vi "4 probe data-osc-time v1.5.vi"() -> ()   [LabVIEW 2014]
uses:
  <vilib>/Analysis/baseanly.llb/Mean (DBL).vi
  <instrlib>/Tektronix TDS 200 1000 2000 Series/Tektronix TDS 200 1000 2000 Series.lvlib
  <vilib>/Analysis/NI_AALBase.lvlib
panel:
  out "Seconds":sgl
  in  "stop button":bool
  in  "loop num":dbl=10000000000.0
  out "Data IV Keithley":string
  in  "Data IV Keithley 2":path=path "c:/myfile.txt"
  out "IV Curve":cluster{dbl[], i32[]}(graph)
  in  "Stop Button":bool
  out "Ch1":dbl
  out "Ch2":dbl
  out "Ch3":dbl
  out "Ch4":dbl
  in  "Channel 4 (3: Channel 4)":u16(ring)=3 items=["Channel 1", "Channel 2", "Channel 3", "Channel 4", "Math", "Reference A", "Reference B", "Reference C", "Reference D"]
  in  "Probe Attenuation 4 (0.1)":dbl=0.1
  in  "Vertical Coupling 4 (1: DC)":u16(ring)=1 items=["AC", "DC", "Ground"]
  in  "Channel 3 (2: Channel 3)":u16(ring)=2 items=["Channel 1", "Channel 2", "Channel 3", "Channel 4", "Math", "Reference A", "Reference B", "Reference C", "Reference D"]
  in  "Probe Attenuation 3 (0.1)":dbl=0.1
  in  "Vertical Coupling 3 (1: DC)":u16(ring)=1 items=["AC", "DC", "Ground"]
  in  "Channel 2 (1: Channel 2)":u16(ring)=1 items=["Channel 1", "Channel 2", "Channel 3", "Channel 4", "Math", "Reference A", "Reference B", "Reference C", "Reference D"]
  in  "Channel 1 (0: Channel 1)":u16(ring) items=["Channel 1", "Channel 2", "Channel 3", "Channel 4", "Math", "Reference A", "Reference B", "Reference C", "Reference D"]
  in  "Serial Configuration":T1={"Baud Rate"=9600, "Parity"=0, "Stop Bits"=10, "Flow Control"=2} {"Flow Control" items=["None", "XON/XOFF", "RTS/CTS", "XON/XOFF & RTS/CTS", "DTR/DSR", "XON/XOFF & DTR/DSR"]; "Stop Bits" items=["1.0"=10, "1.5"=15, "2.0"=20]; "Parity" items=["None", "Odd", "Even", "Mark", "Space"]; "Baud Rate" items=["300"=300, "600"=600, "1200"=1200, "2400"=2400, "4800"=4800, "9600"=9600, "19200"=19200]}
  in  "Probe Attenuation 2 (0.1)":dbl=0.1
  in  "Vertical Coupling 2 (1: DC)":u16(ring)=1 items=["AC", "DC", "Ground"]
  in  "Probe Attenuation 1 (0.1)":dbl=0.1
  in  "Vertical Coupling 1 (1: DC)":u16(ring)=1 items=["AC", "DC", "Ground"]
  in  "Timeout (10000 ms)":u32=500
  in  "VISA resource name":refnum<visa-resource-name>="USB0::0x0699::0x03A6::C044157::INSTR"
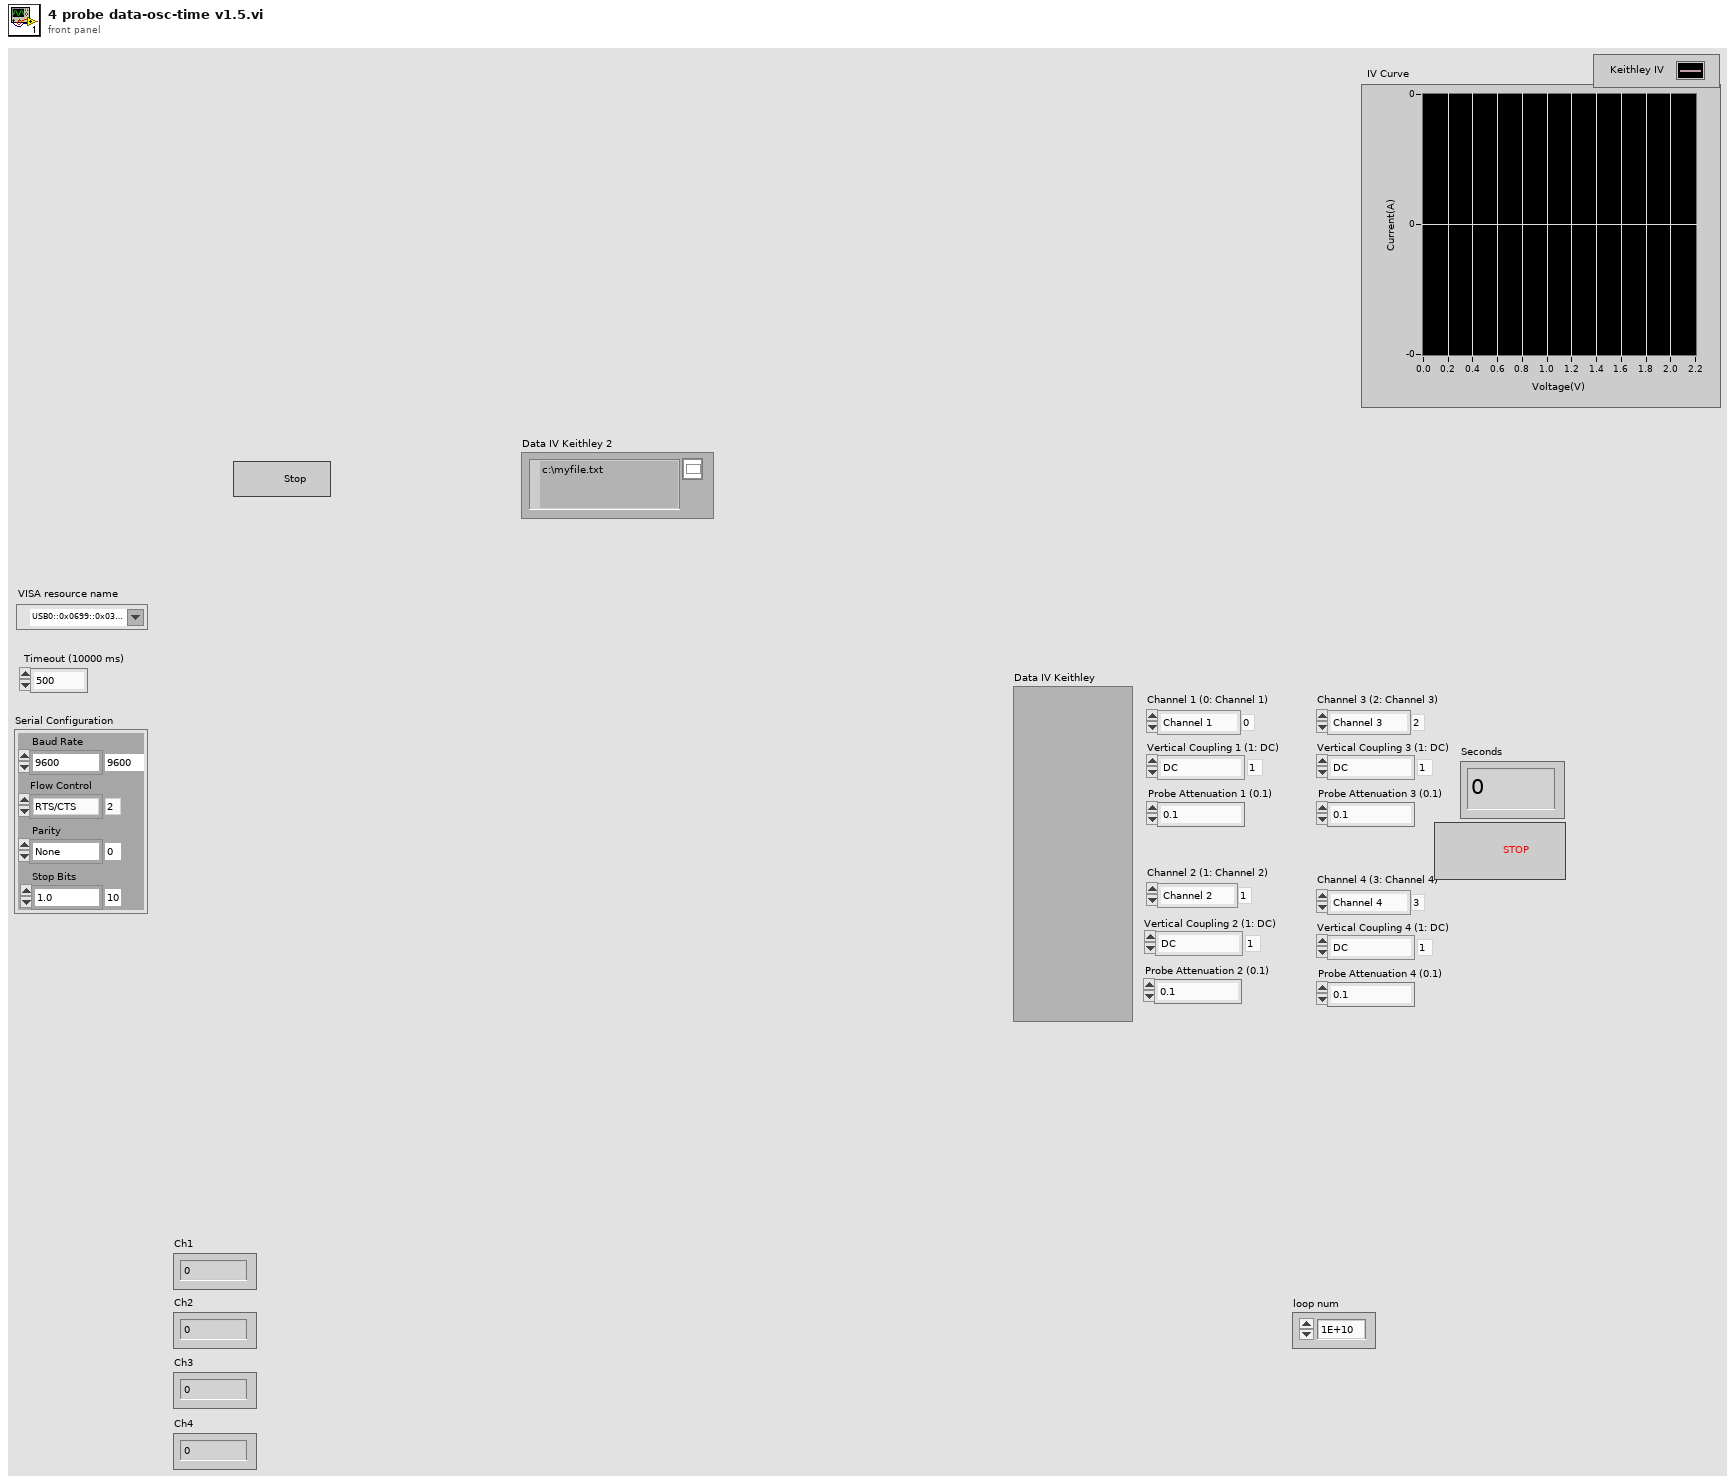
[diagram p1: front panel]
types:
  T1 = cluster{"Baud Rate":u32, "Parity":u16, "Stop Bits":u16, "Flow Control":u16}
  T2 = enum16{"open", "replace", "create", "open or create", "replace or create", "replace or create with confirmation"}
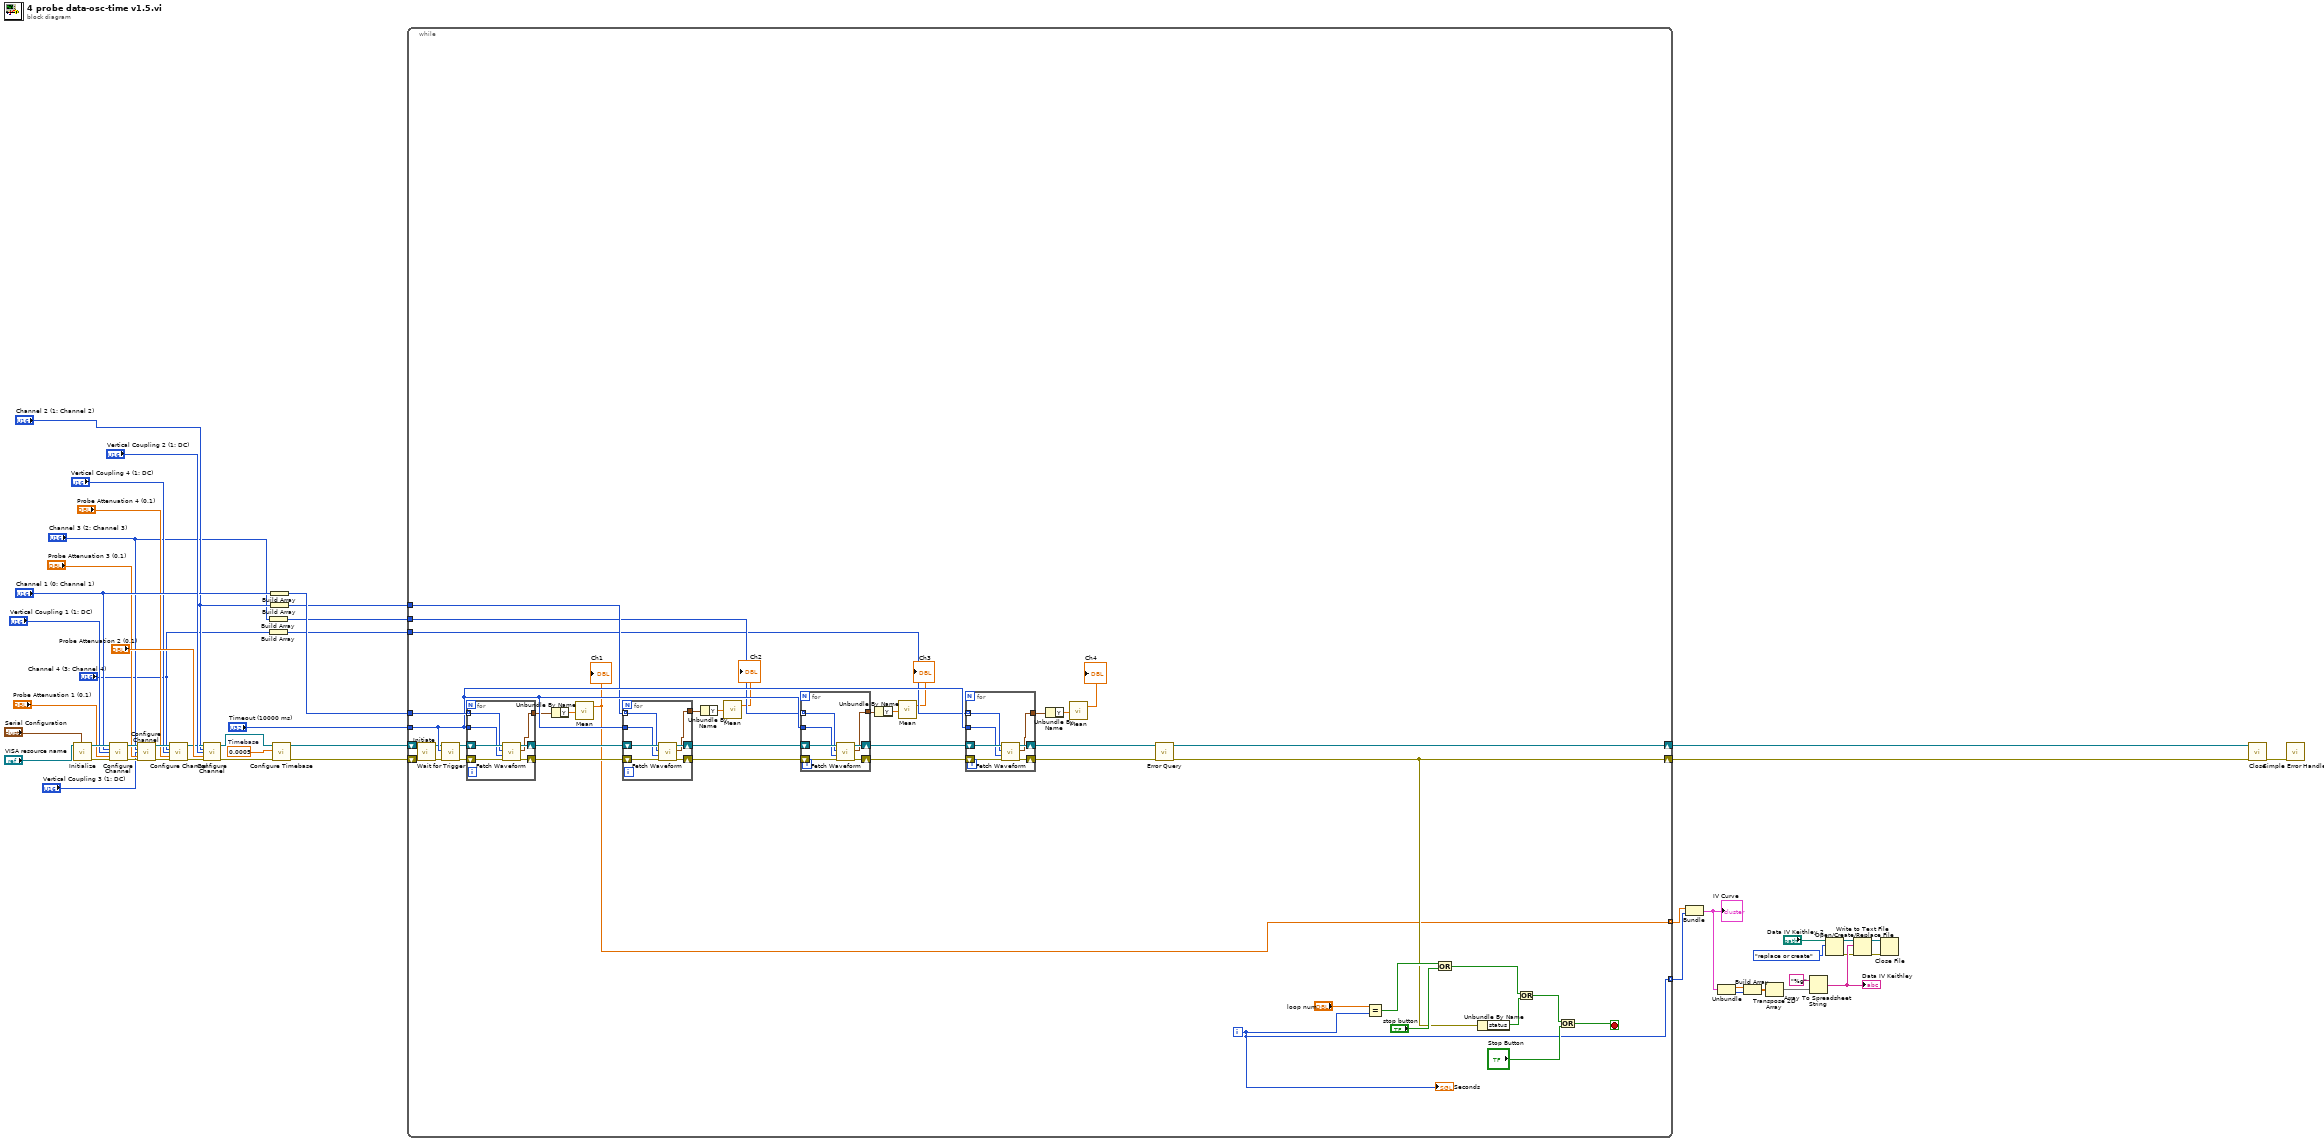
[diagram p0: block diagram]
diagram:
  w36 = 0.0005  # Timebase
  n1 = call <instrlib>:"Initialize.vi"("Serial Configuration"="Serial Configuration", "VISA resource name"="VISA resource name") -> ("error out"=w45:errorcluster, "VISA resource name out"=w46:refnum<visa-resource-name>)  [unwired: 3 in, 5 out]
  n2 = call <instrlib>:"Configure Channel.vi"("VISA resource name"=w46, "Channel (0: Channel 1)"="Channel 1 (0: Channel 1)", "Vertical Coupling (1: DC)"="Vertical Coupling 1 (1: DC)", "Probe Attenuation (10: 10X)"="Probe Attenuation 1 (0.1)", "error in (no error)"=w45) -> ("VISA resource name out"=w31:refnum<visa-resource-name>, "error out"=w28:errorcluster)  [unwired: 4 in, 5 out]
  n3 = call <instrlib>:"Configure Channel.vi"("VISA resource name"=w31, "Channel (0: Channel 1)"="Channel 3 (2: Channel 3)", "Vertical Coupling (1: DC)"="Vertical Coupling 3 (1: DC)", "Probe Attenuation (10: 10X)"="Probe Attenuation 3 (0.1)", "error in (no error)"=w28) -> ("VISA resource name out"=w30:refnum<visa-resource-name>, "error out"=w27:errorcluster)  [unwired: 4 in, 5 out]
  n4 = call <instrlib>:"Configure Channel.vi"("VISA resource name"=w30, "Channel (0: Channel 1)"="Channel 4 (3: Channel 4)", "Vertical Coupling (1: DC)"="Vertical Coupling 4 (1: DC)", "Probe Attenuation (10: 10X)"="Probe Attenuation 4 (0.1)", "error in (no error)"=w27) -> ("VISA resource name out"=w29:refnum<visa-resource-name>, "error out"=w26:errorcluster)  [unwired: 4 in, 5 out]
  n5 = call <instrlib>:"Configure Channel.vi"("VISA resource name"=w29, "Channel (0: Channel 1)"="Channel 2 (1: Channel 2)", "Vertical Coupling (1: DC)"="Vertical Coupling 2 (1: DC)", "Probe Attenuation (10: 10X)"="Probe Attenuation 2 (0.1)", "error in (no error)"=w26) -> ("VISA resource name out"=w44:refnum<visa-resource-name>, "error out"=w43:errorcluster)  [unwired: 4 in, 5 out]
  n6 = Build Array("Channel 3 (2: Channel 3)") -> (w17:u16[])
  n7 = Build Array("Channel 4 (3: Channel 4)") -> (w16:u16[])
  n8 = Build Array("Channel 1 (0: Channel 1)") -> (w35:u16[])
  n9 = Build Array("Channel 2 (1: Channel 2)") -> (w20:u16[])
  n10 = call <instrlib>:"Configure Timebase.vi"("error in (no error)"=w43, "Timebase (0.0005 s)"=w36, "VISA resource name"=w44) -> ("error out"=w41:errorcluster, "VISA resource name out"=w42:refnum<visa-resource-name>)  [unwired: 1 in, 6 out]
  n11 = while {
    tunnel: w35 -> [w89]
    tunnel: "Timeout (10000 ms)" -> [w88]
    tunnel: w20 -> [w87]
    tunnel: w17 -> [w86]
    tunnel: w16 -> [w85]
    shift-right: [w92] -> w48
    shift-left: w42 -> [w91]
    shift-right: [w56] -> w47
    shift-left: w41 -> [w90]
    tunnel: [w52] -> w2 mode=indexing
    tunnel: [w51] -> w1 mode=indexing
    i -> [w52]
    stop <- w53 stop-if-true
    n12 = call <instrlib>:"Initiate.vi"("error in (no error)"=w90, "VISA resource name"=w91) -> ("error out"=w81:errorcluster, "VISA resource name out"=w84:refnum<visa-resource-name>)  [unwired: 8 out]
    n13 = call <instrlib>:"Wait for Trigger.vi"("error in (no error)"=w81, "Timeout (10000 ms)"=w88, "VISA resource name"=w84) -> ("error out"=w82:errorcluster, "VISA resource name out"=w83:refnum<visa-resource-name>)  [unwired: 7 out]
    n14 = for {
      shift-right: [w119] -> w79
      shift-left: w82 -> [w117]
      tunnel: w89 -> [w115] mode=indexing
      tunnel: w88 -> [w116]
      shift-right: [w120] -> w80
      shift-left: w83 -> [w118]
      tunnel: [w114] -> w72
      n15 = call <instrlib>:"Fetch Waveform.vi"("error in (no error)"=w117, "Timeout (10000 ms)"=w116, "Source (0: Channel 1)"=w115, "VISA resource name"=w118) -> ("error out"=w119:errorcluster, "Waveform Data"=w114:waveform(dbl), "VISA resource name out"=w120:refnum<visa-resource-name>)  [unwired: 2 in, 3 out]
    }
    n16 = Unbundle By Name(w72) -> ("Y"=w71:dbl[])
    n17 = call-poly <vilib>:"Mean.vi"("X"=w71) -> ("mean"=w51:dbl)  [unwired: 1 out]
    "Ch1" <- w51
    n18 = for {
      shift-right: [w112] -> w73
      shift-left: w79 -> [w110]
      tunnel: w87 -> [w108] mode=indexing
      tunnel: w88 -> [w109]
      shift-right: [w113] -> w74
      shift-left: w80 -> [w111]
      tunnel: [w107] -> w68
      n19 = call <instrlib>:"Fetch Waveform.vi"("error in (no error)"=w110, "Timeout (10000 ms)"=w109, "Source (0: Channel 1)"=w108, "VISA resource name"=w111) -> ("error out"=w112:errorcluster, "Waveform Data"=w107:waveform(dbl), "VISA resource name out"=w113:refnum<visa-resource-name>)  [unwired: 2 in, 3 out]
    }
    n20 = Unbundle By Name(w68) -> ("Y"=w67:dbl[])
    n21 = call-poly <vilib>:"Mean.vi"("X"=w67) -> ("mean"=→"Ch2":dbl)  [unwired: 1 out]
    n22 = for {
      shift-right: [w105] -> w77
      shift-left: w73 -> [w103]
      tunnel: w86 -> [w101] mode=indexing
      tunnel: w88 -> [w102]
      shift-right: [w106] -> w78
      shift-left: w74 -> [w104]
      tunnel: [w100] -> w69
      n23 = call <instrlib>:"Fetch Waveform.vi"("error in (no error)"=w103, "Timeout (10000 ms)"=w102, "Source (0: Channel 1)"=w101, "VISA resource name"=w104) -> ("error out"=w105:errorcluster, "Waveform Data"=w100:waveform(dbl), "VISA resource name out"=w106:refnum<visa-resource-name>)  [unwired: 2 in, 3 out]
    }
    n24 = Unbundle By Name(w69) -> ("Y"=w66:dbl[])
    n25 = call-poly <vilib>:"Mean.vi"("X"=w66) -> ("mean"=→"Ch3":dbl)  [unwired: 1 out]
    n26 = for {
      shift-right: [w98] -> w75
      shift-left: w77 -> [w96]
      tunnel: w85 -> [w94] mode=indexing
      tunnel: w88 -> [w95]
      shift-right: [w99] -> w76
      shift-left: w78 -> [w97]
      tunnel: [w93] -> w70
      n27 = call <instrlib>:"Fetch Waveform.vi"("error in (no error)"=w96, "Timeout (10000 ms)"=w95, "Source (0: Channel 1)"=w94, "VISA resource name"=w97) -> ("error out"=w98:errorcluster, "Waveform Data"=w93:waveform(dbl), "VISA resource name out"=w99:refnum<visa-resource-name>)  [unwired: 2 in, 3 out]
    }
    n28 = Unbundle By Name(w70) -> ("Y"=w65:dbl[])
    n29 = call-poly <vilib>:"Mean.vi"("X"=w65) -> ("mean"=→"Ch4":dbl)  [unwired: 1 out]
    n30 = call <instrlib>:"Error Query.vi"("error in (no error)"=w75, "VISA resource name"=w76) -> ("error out"=w56:errorcluster, "VISA resource name out"=w92:refnum<visa-resource-name>)  [unwired: 8 out]
    n31 = Equal?(x="loop num", y=w52) -> (x = y?=w57:bool)
    n32 = Or(x=w57, y="stop button") -> (x .or. y?=w58:bool)
    n33 = Unbundle By Name(w56) -> ("status"=w59:bool)
    n34 = Or(x=w58, y=w59) -> (x .or. y?=w55:bool)
    n35 = Or(x=w55, y="Stop Button") -> (x .or. y?=w53:bool)
    "Seconds" <- w52
  }
  n36 = Bundle(w1, w2) -> (w9:cluster{dbl[], i32[]})  [unwired: 1 out]
  "IV Curve" <- w9
  n37 = Unbundle(w9) -> (w10:dbl[], w11:i32[])
  n38 = Build Array(w10, w11) -> (w12:dbl[][])
  n39 = Transpose 2D Array(2D array=w12) -> (transposed array=w14:dbl[][])
  n40 = Array To Spreadsheet String(array=w14, 3:"%g" ("format string")) -> (spreadsheet string=w15:string)  [unwired: 1 in]
  "Data IV Keithley" <- w15
  n41 = Open/Create/Replace File(file path (use dialog)="Data IV Keithley 2", operation (0:open)=T2."replace or create") -> (refnum out=w8:refnum<file>, error out=w3:errorcluster)  [unwired: 4 in, 1 out]
  n42 = Write to Text File(file (use dialog)=w8, text=w15, error in=w3) -> (refnum out=w5:refnum<file>, error out=w4:errorcluster)  [unwired: 2 out]
  n43 = Close File(refnum=w5, error in=w4) -> ()  [unwired: 2 out]
  n44 = call <instrlib>:"Close.vi"("error in (no error)"=w47, "VISA resource name"=w48) -> ("error out"=w49:errorcluster)  [unwired: 9 out]
  n45 = call <vilib>:"Simple Error Handler.vi"("error in (no error)"=w49) -> ()  [unwired: 1 in, 8 out]
